vi "State Machine Kernel.vi"(4 "Init?":bool, 5 "Inputs":T3, 6 "StateData":T1, 7 "Stop":bool) -> (0 "Terminated?":bool, 1 "Outputs":T2, 2 "StateData":T1)   [LabVIEW 2017]
uses:
  Controls/Inputs.ctl
  Controls/Outputs.ctl
  <vilib>/myRIO/Instrument Drivers/Onboard IO/PWM/typedefs/PWM Reference.ctl
  <vilib>/myRIO/Common/Instrument Driver Framework/Utilities/typedefs/myRIO Generic Hardware Reference.ctl
  <vilib>/myRIO/Common/Instrument Driver Framework/Utilities/typedefs/Hardware Version Enum.ctl
  <vilib>/myRIO/Common/Instrument Driver Framework/Utilities/typedefs/myRIO v1.0 Reference.ctl
  <vilib>/myRIO/Common/Instrument Driver Framework/Utilities/typedefs/Generic FPGA Reference.ctl
  <vilib>/myRIO/Common/Instrument Driver Framework/myRIO v1.0/PWM/typedefs/PWM Channels Enum.ctl
  <vilib>/myRIO/Instrument Drivers/Onboard IO/PWM/typedefs/PWM Configuration.ctl
  <vilib>/userdefined/High Color/nirio_resource_hc.ctl
  <vilib>/myRIO/Common/Instrument Driver Framework/Utilities/vis/Is FPGA Ref Available.vi
  <vilib>/myRIO/Common/Instrument Driver Framework/myRIO v1.0/PWM/vis/myRIO v1.1 Open PWM.vi
  <vilib>/myRIO/Instrument Drivers/Onboard IO/PWM/vis/Set Duty Cycle and Frequency.vi
  <vilib>/myRIO/Common/Instrument Driver Framework/Utilities/vis/Validate Channels.vi
  <vilib>/myRIO/Common/Instrument Driver Framework/myRIO v1.0/PWM/vis/myRIO v1.0 Reserve PWM.vi
  <vilib>/myRIO/Common/Instrument Driver Framework/myRIO v1.0/PWM/vis/myRIO v1.0 Build MUX Configuration PWM.vi
  <vilib>/myRIO/Common/Instrument Driver Framework/myRIO v1.0/Resource Manager/vis/myRIO v1.0 Reserve Channel List.vi
  <vilib>/myRIO/Common/Instrument Driver Framework/myRIO v1.0/Resource Manager/vis/myRIO v1.0 Create Configuration List.vi
  <vilib>/myRIO/Common/Instrument Driver Framework/myRIO v1.0/Resource Manager/vis/myRIO v1.0 Reserve Channel.vi
  <vilib>/myRIO/Common/Instrument Driver Framework/myRIO v1.0/Resource Manager/vis/myRIO v1.0 Unreserve Channel.vi
  <vilib>/myRIO/Common/Instrument Driver Framework/myRIO v1.0/Resource Manager/vis/myRIO v1.0 Build Mutex Name.vi
  <vilib>/Utility/VariantDataType/GetNumericInfo.vi
  <vilib>/Utility/error.llb/Error Cluster From Error Code.vi
  <vilib>/myRIO/Common/Instrument Driver Framework/myRIO v1.0/myRIO v1.1 Open.vi
  <vilib>/myRIO/Common/Instrument Driver Framework/Utilities/vis/IO Manager.vi
  <vilib>/myRIO/Common/Instrument Driver Framework/Utilities/vis/Configuration Manager.vi
  <vilib>/myRIO/Common/Instrument Driver Framework/myRIO v1.0/Resource Manager/vis/myRIO v1.0 Configure IO.vi
  <vilib>/myRIO/Common/Instrument Driver Framework/myRIO v1.0/myRIO v1.0 Close.vi
  <vilib>/myRIO/Common/Instrument Driver Framework/myRIO v1.0/PWM/vis/myRIO v1.0 Write PWM.vi
  <vilib>/myRIO/Express VI/Onboard IO/PWM/PWM Express VI.xnode
  <vilib>/myRIO/Instrument Drivers/Onboard IO/PWM/vis/myRIO PWM Open.xnode
  <vilib>/myRIO/Instrument Drivers/Onboard IO/PWM/PWM.lvlib
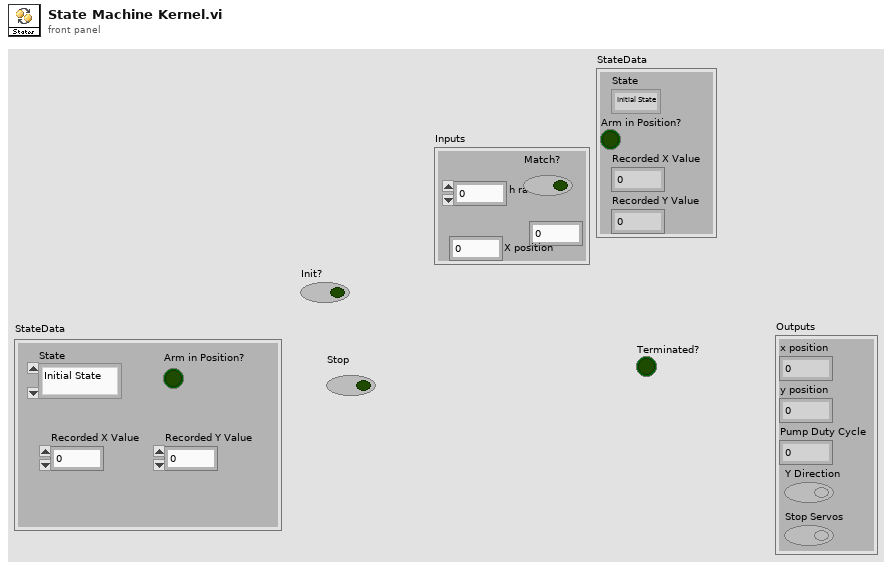
[diagram p1: front panel]
types:
  T1 = cluster{"State":enum16{"Initial State", "Pre Move", "Move Arm", "Fill Water"}, "Arm in Position?":bool, "Recorded X Value":dbl, "Recorded Y Value":dbl}
  T2 = typedef "Outputs.ctl" = cluster{"x position":dbl, "y position":dbl, "Pump Duty Cycle":dbl, "Y Direction":bool, "Stop Servos":bool}
  T3 = typedef "Inputs.ctl" = cluster{"X position":dbl, "Y position":dbl, "h ratio":dbl, "Match?":bool}
  T4 = enum16{"Initial State", "Pre Move", "Move Arm", "Fill Water"}
  T5 = typedef "PWM.lvlib/PWM Reference.ctl" = cluster{"myRIO Reference":T6, "PWM Channels Enum":T10, "PWM Configuration":T11}
  T6 = typedef "myRIO Generic Hardware Reference.ctl" = cluster{"myRIO Model":T7, "myRIO Hardware Reference":T8}
  T7 = typedef "Hardware Version Enum.ctl" = enum16{"Unknown", "myRIO-1900", "myRIO-1950", "roboRIO", "NI ELVIS RIO CM"}
  T8 = typedef "myRIO v1.0 Reference.ctl" = cluster{"Generic FPGA Reference":T9, "Allow multiple opens":bool}
  T9 = typedef "Generic FPGA Reference.ctl" = refnum<k20>
  T10 = typedef "PWM Channels Enum.ctl" = enum16{"Not Connected", "C/PWM0", "C/PWM1", "A/PWM0", "A/PWM1", "A/PWM2", "B/PWM0", "B/PWM1", "B/PWM2", "PWM/PWM0", "PWM/PWM1", "PWM/PWM2", "PWM/PWM3", "PWM/PWM4", "PWM/PWM5", "PWM/PWM6", "PWM/PWM7", "PWM/PWM8", "PWM/PWM9"}
  T11 = typedef "PWM.lvlib/PWM Configuration.ctl" = cluster{"Frequency":dbl, "Duty Cycle":dbl}
  T12 = typedef "nirio_resource_hc.ctl" = tag
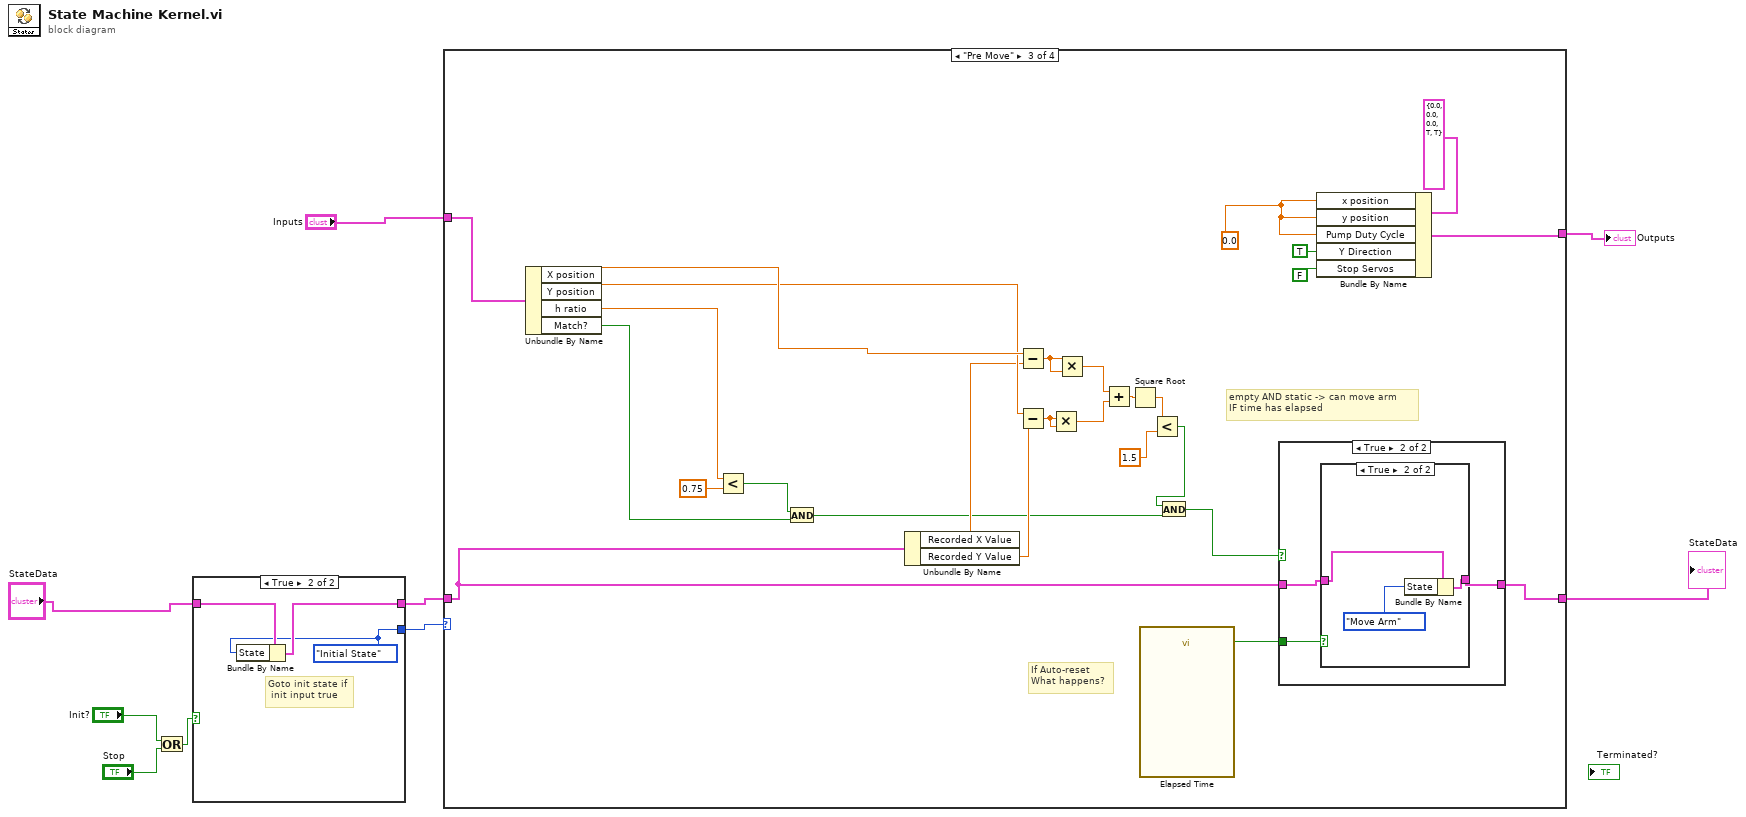
[diagram p0: block diagram]
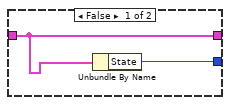
[diagram p2: hidden frame]
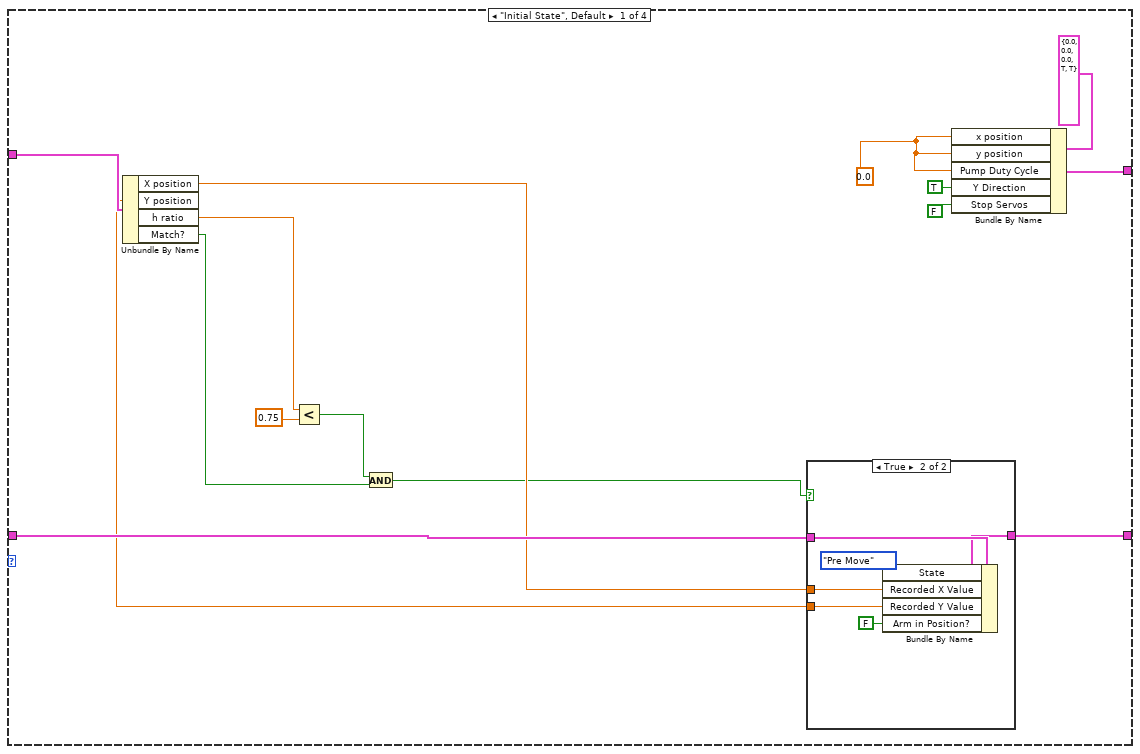
[diagram p3: hidden frame]
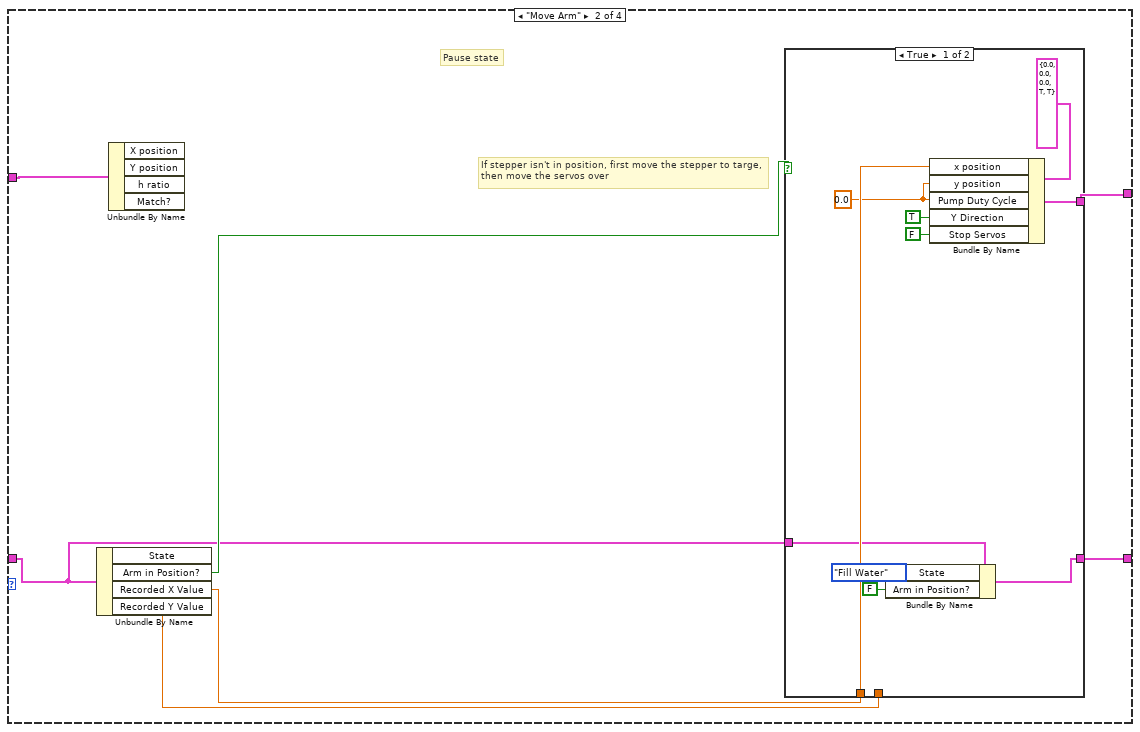
[diagram p5: hidden frame]
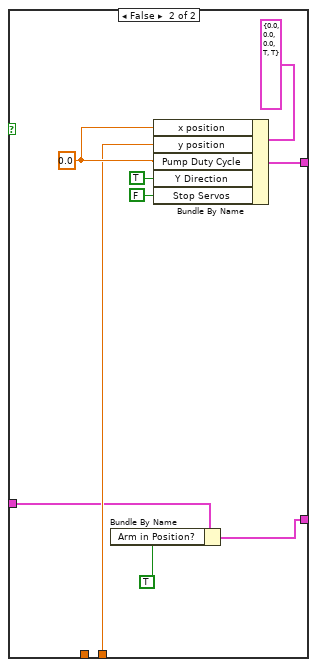
[diagram p6: hidden frame]
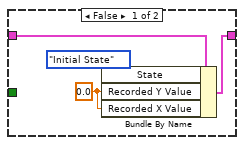
[diagram p7: hidden frame]
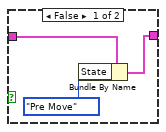
[diagram p8: hidden frame]
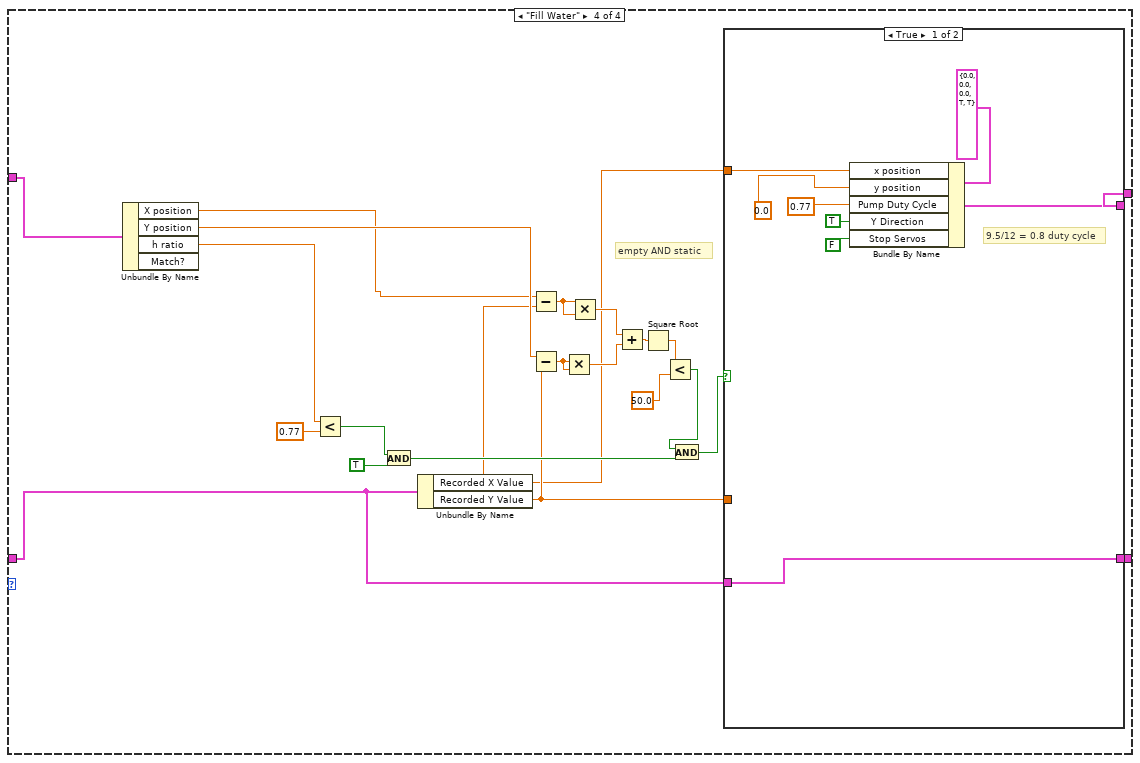
[diagram p9: hidden frame]
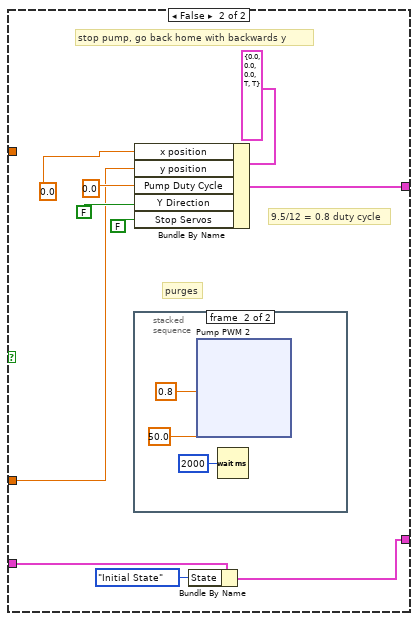
[diagram p10: hidden frame]
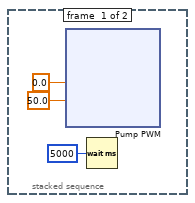
[diagram p11: hidden frame]
diagram:
  n1 = Or(x="Init?", y="Stop") -> (x .or. y?=w1:bool)
  n2 = case shown="True" w1 {
    tunnel: "StateData" -> [w11 w14]
    tunnel: [w11 w13] -> w7
    tunnel: [w10 w12] -> w4
    frame False {
      n3 = Unbundle By Name(w11) -> ("State"=w10:T4)
    }
    frame True {
      w12 = T4."Initial State" ("State")
      # "Goto init state if\n init input true"
      n4 = Bundle By Name(cluster=w14, "State"=w12) -> (w13:T1)
    }
  }
  n5 = case shown="\"Pre Move\"" w4 {
    tunnel: "Inputs" -> [w29 w42 w89 w111]
    tunnel: [w25 w43 w71 w109] -> w8
    tunnel: w7 -> [w23 w38 w87 w108]
    tunnel: [w24 w37 w88 w107] -> w6
    frame "Initial State", Default {
      w27 = 0.0
      n6 = Unbundle By Name(w29) -> ("X position"=w22:dbl, "Y position"=w21:dbl, "h ratio"=w17:dbl, "Match?"=w20:bool)
      n7 = Less?(x=w17, y=0.75) -> (x < y?=w16:bool)
      n8 = And(x=w16, y=w20) -> (x .and. y?=w19:bool)
      n9 = case shown="True" w19 {
        tunnel: w23 -> [w30 w36]
        tunnel: [w30 w35] -> w24
        tunnel: w22 -> [_ w33]
        tunnel: w21 -> [_ w32]
        frame False {
        }
        frame True {
          n10 = Bundle By Name(cluster=w36, "State"=T4."Pre Move", "Recorded X Value"=w33, "Recorded Y Value"=w32, "Arm in Position?"=FALSE) -> (w35:T1)
        }
      }
      n11 = Bundle By Name(cluster=T2 {"x position"=0.0, "y position"=0.0, "Pump Duty Cycle"=0.0, "Y Direction"=TRUE, "Stop Servos"=TRUE} ("Outputs"), "x position"=w27, "y position"=w27, "Pump Duty Cycle"=w27, "Y Direction"=TRUE, "Stop Servos"=FALSE) -> (w25:T2)
    }
    frame "Move Arm" {
      # "If stepper isn't in position, first move the stepper to targe, then move the servos over"
      # "Pause state"
      n12 = Unbundle By Name(w38) -> ("Arm in Position?"=w41:bool, "Recorded X Value"=w40:dbl, "Recorded Y Value"=w39:dbl)  [unwired: 1 out]
      n13 = Unbundle By Name(w42) -> ()  [unwired: 4 out]
      n14 = case shown="True" w41 {
        tunnel: [w51 w60] -> w43
        tunnel: w40 -> [w50 _]
        tunnel: w39 -> [_ w58]
        tunnel: w38 -> [w48 w57]
        tunnel: [w47 w56] -> w37
        frame True {
          w49 = 0.0
          n15 = Bundle By Name(cluster=w48, "State"=T4."Fill Water", "Arm in Position?"=FALSE) -> (w47:T1)
          n16 = Bundle By Name(cluster=T2 {"x position"=0.0, "y position"=0.0, "Pump Duty Cycle"=0.0, "Y Direction"=TRUE, "Stop Servos"=TRUE} ("Outputs"), "x position"=w50, "y position"=w49, "Pump Duty Cycle"=w49, "Y Direction"=TRUE, "Stop Servos"=FALSE) -> (w51:T2)
        }
        frame False {
          w59 = 0.0
          n17 = Bundle By Name(cluster=w57, "Arm in Position?"=TRUE) -> (w56:T1)
          n18 = Bundle By Name(cluster=T2 {"x position"=0.0, "y position"=0.0, "Pump Duty Cycle"=0.0, "Y Direction"=TRUE, "Stop Servos"=TRUE} ("Outputs"), "x position"=w59, "y position"=w58, "Pump Duty Cycle"=w59, "Y Direction"=TRUE, "Stop Servos"=FALSE) -> (w60:T2)
        }
      }
    }
    frame "Pre Move" {
      w73 = 0.0
      # "empty AND static -> can move arm\nIF time has elapsed"
      # "If Auto-reset\nWhat happens?"
      n19 = Unbundle By Name(w89) -> ("X position"=w86:dbl, "Y position"=w85:dbl, "h ratio"=w67:dbl, "Match?"=w68:bool)
      n20 = Less?(x=w67, y=0.75) -> (x < y?=w69:bool)
      n21 = And(x=w69, y=w68) -> (x .and. y?=w66:bool)
      n22 = Unbundle By Name(w87) -> ("Recorded X Value"=w84:dbl, "Recorded Y Value"=w83:dbl)
      n23 = Subtract(x=w86, y=w84) -> (x-y=w82:dbl)
      n24 = Subtract(x=w85, y=w83) -> (x-y=w81:dbl)
      n25 = Multiply(x=w81, y=w81) -> (x*y=w79:dbl)
      n26 = Multiply(x=w82, y=w82) -> (x*y=w80:dbl)
      n27 = Add(x=w80, y=w79) -> (x+y=w78:dbl)
      n28 = Square Root(x=w78) -> (sqrt(x)=w76:dbl)
      n29 = call "Elapsed Time"() -> ("Time has Elapsed"=w75:bool)  [unwired: 12 in, 7 out]
      n30 = Less?(x=w76, y=1.5) -> (x < y?=w65:bool)
      n31 = And(x=w65, y=w66) -> (x .and. y?=w64:bool)
      n32 = case shown="True" w64 {
        tunnel: w87 -> [w93 w96]
        tunnel: [w92 w94] -> w88
        tunnel: w75 -> [_ w95]
        frame False {
          w90 = 0.0 ("Recorded Y Value")
          n33 = Bundle By Name(cluster=w93, "State"=T4."Initial State", "Recorded Y Value"=w90, "Recorded X Value"=w90) -> (w92:T1)
        }
        frame True {
          n34 = case shown="True" w95 {
            tunnel: w96 -> [w98 w101]
            tunnel: [w97 w100] -> w94
            frame False {
              n35 = Bundle By Name(cluster=w98, "State"=T4."Pre Move") -> (w97:T1)
            }
            frame True {
              n36 = Bundle By Name(cluster=w101, "State"=T4."Move Arm") -> (w100:T1)
            }
          }
        }
      }
      n37 = Bundle By Name(cluster=T2 {"x position"=0.0, "y position"=0.0, "Pump Duty Cycle"=0.0, "Y Direction"=TRUE, "Stop Servos"=TRUE} ("Outputs"), "x position"=w73, "y position"=w73, "Pump Duty Cycle"=w73, "Y Direction"=TRUE, "Stop Servos"=FALSE) -> (w71:T2)
    }
    frame "Fill Water" {
      # "empty AND static"
      n38 = Unbundle By Name(w111) -> ("X position"=w105:dbl, "Y position"=w124:dbl, "h ratio"=w114:dbl)  [unwired: 1 out]
      n39 = Less?(x=w114, y=0.77) -> (x < y?=w115:bool)
      n40 = And(x=w115, y=TRUE) -> (x .and. y?=w113:bool)
      n41 = Unbundle By Name(w108) -> ("Recorded X Value"=w104:dbl, "Recorded Y Value"=w106:dbl)
      n42 = Subtract(x=w105, y=w104) -> (x-y=w123:dbl)
      n43 = Subtract(x=w124, y=w106) -> (x-y=w122:dbl)
      n44 = Multiply(x=w122, y=w122) -> (x*y=w120:dbl)
      n45 = Multiply(x=w123, y=w123) -> (x*y=w121:dbl)
      n46 = Add(x=w121, y=w120) -> (x+y=w119:dbl)
      n47 = Square Root(x=w119) -> (sqrt(x)=w117:dbl)
      n48 = Less?(x=w117, y=50.0) -> (x < y?=w112:bool)
      n49 = And(x=w112, y=w113) -> (x .and. y?=w110:bool)
      n50 = case shown="True" w110 {
        tunnel: [w129 w139] -> w109
        tunnel: w108 -> [w127 w136]
        tunnel: [w127 w135] -> w107
        tunnel: w106 -> [_ w133]
        tunnel: w104 -> [w126 _]
        frame True {
          # "9.5/12 = 0.8 duty cycle"
          n51 = Bundle By Name(cluster=T2 {"x position"=0.0, "y position"=0.0, "Pump Duty Cycle"=0.0, "Y Direction"=TRUE, "Stop Servos"=TRUE} ("Outputs"), "x position"=w126, "y position"=0.0, "Pump Duty Cycle"=0.77, "Y Direction"=TRUE, "Stop Servos"=FALSE) -> (w129:T2)
        }
        frame False {
          # "purges"
          # "stop pump, go back home with backwards y"
          # "9.5/12 = 0.8 duty cycle"
          n52 = stacked-sequence {
            frame #0 {
              n53 = xnode "Pump PWM"("Duty Cycle"=0.0, "Frequency [Hz]"=50.0) -> ()  [unwired: 1 in, 1 out]
              n54 = Wait (ms)(milliseconds to wait=u32 5000) -> ()  [unwired: 1 out]
            }
            frame #1 {
              n55 = xnode "Pump PWM 2"("Duty Cycle"=0.8, "Frequency [Hz]"=50.0) -> ()  [unwired: 1 in, 1 out]
              n56 = Wait (ms)(milliseconds to wait=u32 2000) -> ()  [unwired: 1 out]
            }
          }
          n57 = Bundle By Name(cluster=T2 {"x position"=0.0, "y position"=0.0, "Pump Duty Cycle"=0.0, "Y Direction"=TRUE, "Stop Servos"=TRUE} ("Outputs"), "x position"=0.0, "y position"=w133, "Pump Duty Cycle"=0.0, "Y Direction"=FALSE, "Stop Servos"=FALSE) -> (w139:T2)
          n58 = Bundle By Name(cluster=w136, "State"=T4."Initial State") -> (w135:T1)
        }
      }
    }
  }
  "Outputs" <- w8
  "StateData" <- w6
